vi "Format TimeStamp Control.vi"(6 "Format String":string, 8 "error in":errorcluster, 11 "GObject in":refnum<vi>) -> (0 "error out":errorcluster, 2 "Successful":bool)   [LabVIEW 2019, in "Quick Format QD.lvlib"]
doc: "Formats a TimeStamp control based on the given Format String."
uses:
  Quick Format QD.lvlib
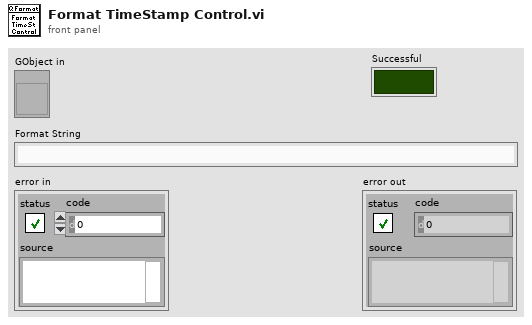
[diagram p1: front panel]
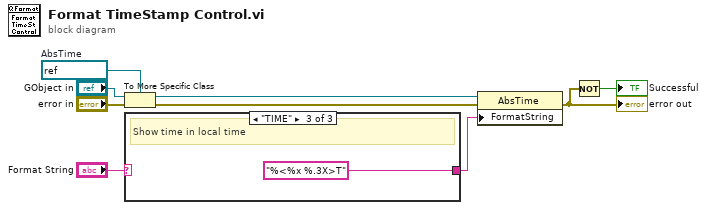
[diagram p0: block diagram]
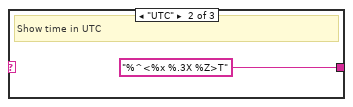
[diagram p3: hidden frame]
diagram:
  w6 = refnum<vi> refnum  # AbsTime
  n1 = To More Specific Class(target class=w6, reference="GObject in", error in="error in") -> (specific class reference=w2:refnum<vi>, error out=w8:errorcluster)
  n2 = case shown="\"TIME\"" "Format String" {
    selector: "Format String" -> [w10 _ _]
    tunnel: [w10 "%^<%x %.3X %Z>T" "%<%x %.3X>T"] -> w1
    frame Default {
      # "Custom Format String.  Write FormatString directly."
    }
    frame "UTC" {
      # "Show time in UTC"
    }
    frame "TIME" {
      # "Show time in local time"
    }
  }
  n3 = property on="Property Node" class="AbsTime"(reference=w2, error in=w8, "FormatString"=w1) -> (error out=w7:errorcluster)  [unwired: 1 out]
  "error out" <- w7
  n4 = Not(x=w7) -> (.not. x?=→"Successful":bool)
